vi "Create.vi"(9 "Alias":string, 10 "Actor":refnum<class "Actor.lvclass">, 11 "Ex Event Actor in":refnum<class "Ex Event Actor.lvclass">) -> (3 "Ex Event Actor out":refnum<class "Ex Event Actor.lvclass">)   [LabVIEW 2021, in "Ex Event Actor.lvclass"]
uses:
  Ex Event Actor.lvclass
  Actor/Actor/Actor.lvclass
  Ex Event Actor.lvclass/Ex Event Actor.ctl
  Actor/Event Actor/Event Actor.lvclass
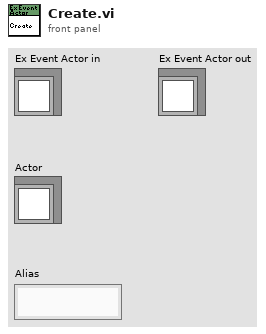
[diagram p1: front panel]
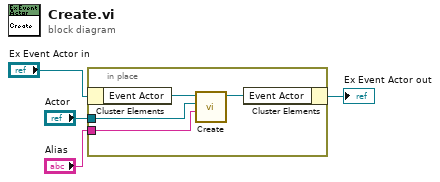
[diagram p0: block diagram]
diagram:
  n1 = in-place {
    in-place-border: "Actor" -> [w6]
    in-place-border: "Alias" -> [w5]
    n2 = in-place-cluster #1("Ex Event Actor in") -> ("Event Actor"=w8:refnum<class "Event Actor.lvclass">)
    n3 = call-dynamic "Create.vi"("Alias"=w5, "Actor"=w6, "Create in"=w8) -> ("Create out"=w7:refnum<class "Event Actor.lvclass">)  [unwired: 8 in]
    n4 = in-place-cluster #1("Event Actor"=w7) -> (→"Ex Event Actor out":refnum<class "Ex Event Actor.lvclass">)
  }
